vi "dangerEnemy.vi"(8 "error in (no error)":errorcluster, 10 "Game":refnum<class "Game.lvclass">, 11 "Utilities in":refnum<class "Utilities.lvclass">) -> (0 "error out":errorcluster, 2 "Id do Inimigo Mais Próximo":u32, 3 "Utilities out":refnum<class "Utilities.lvclass">, 4 "id do segundo inimigo mais perigoso":i32, 5 "id do inimigo\nmais perigoso":i32, 6 "Pos do segundo inimigo\nperigoso":dbl[](array[numeric]), 7 "Pos do inimigo\nmais perigoso":dbl[](array[numeric]))   [LabVIEW 2018, in "Utilities.lvclass"]
uses:
  Utilities.lvclass
  Game_class/Game.lvclass
  Game_class/Game.lvclass/Game.ctl
  Referee_class/Referee.lvclass/Referee.ctl
  Team_class/Team.lvclass/Team.ctl
  Object_class/Object.lvclass/Object.ctl
  Robot_class/Robot.lvclass/Robot.ctl
  Object_class/Read x.vi
  Object_class/Read y.vi
  Robot_class/Read id.vi
  <vilib>/Analysis/_algsub.llb/Real Vector Norm.vi
  Game_class/Read Referee.vi
  Game_class/Read FieldRef.vi
  Game_class/Read EnemyRef.vi
  Game_class/Read BallRef.vi
  Team_class/Read RobotRef.vi
  Referee_class/Read enemy_goalie_id.vi
  Enemy_class/Enemy.lvclass
  C:/Users/Ronaldo/Desktop/Phoenix/SSL_AI/Team_class/Team.lvclass
  Ball_class/Ball.lvclass
  C:/Users/Ronaldo/Desktop/Phoenix/SSL_AI/Object_class/Object.lvclass
  Robot_class/Robot.lvclass
  Referee_class/Referee.lvclass
  Field_class/Field.lvclass
  <vilib>/Analysis/NI_AALPro.lvlib
panel:
  out "Numero de inimigos\npossiveis para marcar":i32
  in  "D para nao marcar":dbl=200.0
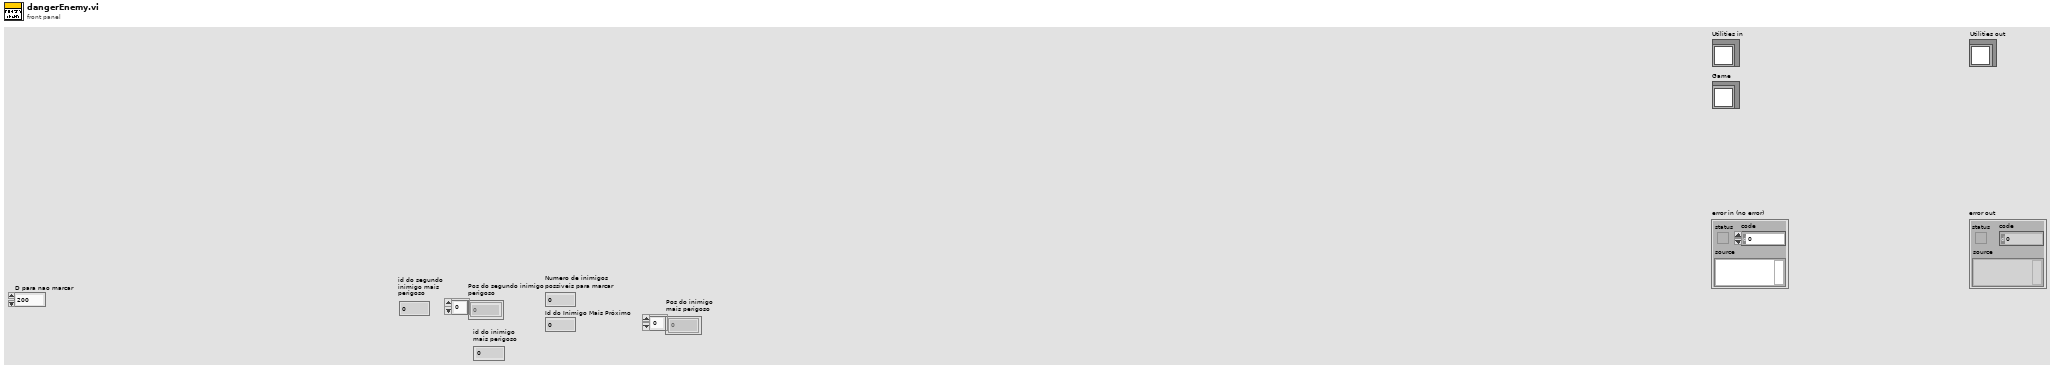
[diagram p1: front panel]
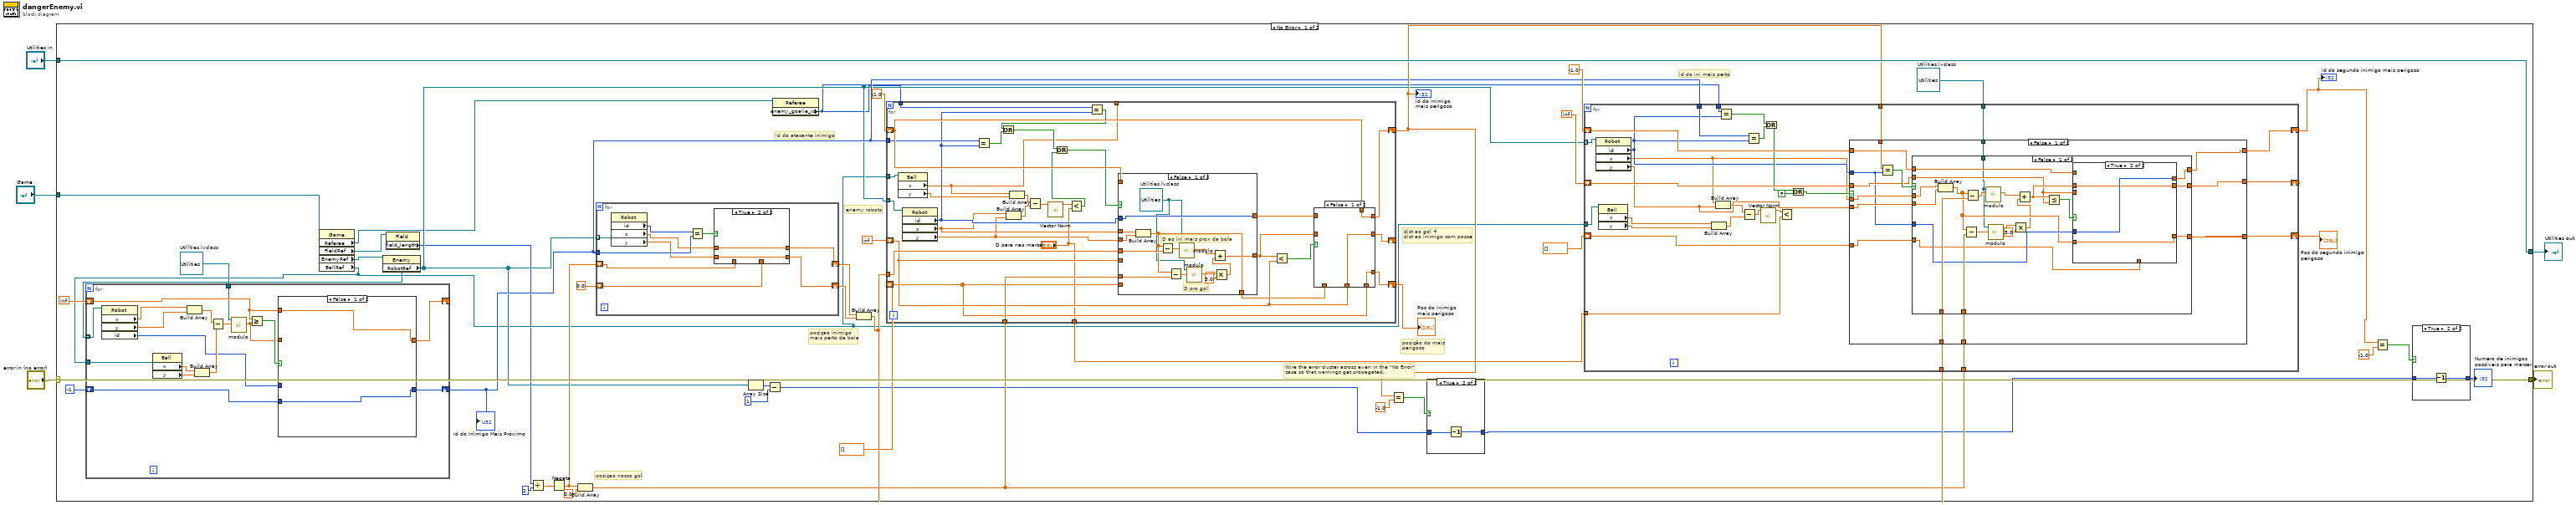
[diagram p0: block diagram]
diagram:
  n1 = case shown="No Error" "error in (no error)" {
    selector: "error in (no error)" -> [w48 w222]
    tunnel: [w48 w222] -> w4
    tunnel: [w49 w221] -> w2
    tunnel: "Utilities in" -> [w49 w221]
    tunnel: "Game" -> [w13 _]
    frame No Error {
      w14 = refnum<class "Utilities.lvclass"> refnum  # Utilities.lvclass
      w15 = refnum<class "Utilities.lvclass"> refnum  # Utilities.lvclass
      # "id do ini mais perto"
      # "id do atacante inimigo"
      # "enemy robots"
      # "dist ao gol +\ndist ao inimigo com posse"
      # "posição do mais\nperigoso"
      # "posiçao nosso gol"
      # "posiçao inimigo\nmais perto da bola"
      # "Wire the error cluster across even in the \"No Error\"\ncase so that warnings get propagated."
      n2 = property class="Game"(reference=w13) -> ("Referee"=w7:refnum<class "Referee.lvclass">, "FieldRef"=w9:refnum<class "Field.lvclass">, "EnemyRef"=w12:refnum<class "Enemy.lvclass">, "BallRef"=w10:refnum<class "Ball.lvclass">)  [unwired: 1 in, 2 out]
      n3 = property class="Enemy"(reference=w12) -> ("RobotRef"=w11:refnum<class "Robot.lvclass">[])  [unwired: 1 in, 2 out]
      n4 = for {
        shift-right: [w67] -> _
        shift-left: inf -> [w65]
        shift-right: [w66] -> w17
        shift-left: -1 -> [w64]
        tunnel: w15 -> [w63]
        tunnel: w10 -> [w62]
        tunnel: w11 -> [w59] mode=indexing
        n5 = property class="Robot"(reference=w59) -> ("x"=w58:dbl, "y"=w57:dbl, "id"=w56:i32)  [unwired: 1 in, 2 out]
        n6 = property class="Ball"(reference=w62) -> ("x"=w61:dbl, "y"=w60:dbl)  [unwired: 1 in, 2 out]
        n7 = Build Array(w58, w57) -> (w72:dbl[])
        n8 = Build Array(w61, w60) -> (w71:dbl[])
        n9 = Subtract(x=w72, y=w71) -> (x-y=w69:dbl[])
        n10 = call "modulo.vi"("2D vector"=w69, "Utilities in"=w63) -> ("Modulo"=w68:dbl)  [unwired: 7 in, 2 out]
        n11 = Greater Or Equal?(x=w65, y=w68) -> (x >= y?=w70:bool)
        n12 = case shown="False" w70 {
          tunnel: [w74 w76] -> w67
          tunnel: w68 -> [_ w76]
          tunnel: w56 -> [_ w75]
          tunnel: [w73 w75] -> w66
          tunnel: w65 -> [w74 _]
          tunnel: w64 -> [w73 _]
          frame False {
          }
          frame True {
          }
        }
      }
      "Id do Inimigo Mais Próximo" <- w17
      n13 = property class="Field"(reference=w9) -> ("field_length"=w8:i32)  [unwired: 1 in, 2 out]
      n14 = Divide(x=w8, y=u32 2) -> (x/y=w45:dbl)
      n15 = Negate(x=w45) -> (-x=w40:dbl)
      n16 = Build Array(w40, 0.0 ("element")) -> (w34:dbl[])
      n17 = for {
        tunnel: w11 -> [w210] mode=indexing
        tunnel: w17 -> [w216]
        shift-right: [w214] -> w19
        shift-left: w40 -> [w212]
        shift-right: [w213] -> w47
        shift-left: 0.0 ("y") -> [w211]
        n18 = property class="Robot"(reference=w210) -> ("id"=w209:i32, "x"=w208:dbl, "y"=w207:dbl)  [unwired: 1 in, 2 out]
        n19 = Equal?(x=w209, y=w216) -> (x = y?=w215:bool)
        n20 = case shown="True" w215 {
          tunnel: w208 -> [_ w220]
          tunnel: w207 -> [_ w219]
          tunnel: [w218 w220] -> w214
          tunnel: [w217 w219] -> w213
          tunnel: w212 -> [w218 _]
          tunnel: w211 -> [w217 _]
          frame False {
          }
          frame True {
          }
        }
      }
      n21 = Array Size(array=w11) -> (size(s)=w31:i32)
      n22 = Subtract(x=w31, y=1) -> (x-y=w26:i32)
      n23 = property class="Referee"(reference=w7) -> ("enemy_goalie_id"=w6:i32)  [unwired: 1 in, 2 out]
      n24 = Build Array(w19, w47) -> (w35:dbl[])
      n25 = for {
        tunnel: w35 -> [w183]
        tunnel: w34 -> [w182]
        shift-right: [w179] -> _
        shift-left: inf -> [w178]
        shift-right: [w176] -> w29
        shift-left: -1.0 ("id") -> [w173]
        shift-right: [w174] -> w43
        shift-left: dbl[] [] -> [w172]
        tunnel: w6 -> [w171]
        tunnel: [w154] -> _
        tunnel: ["D para nao marcar"] -> w20
        tunnel: w17 -> [w161]
        tunnel: w11 -> [w159] mode=indexing
        tunnel: w10 -> [w155]
        n26 = property class="Ball"(reference=w155) -> ("x"=w154:dbl, "y"=w153:dbl)  [unwired: 1 in, 2 out]
        n27 = property class="Robot"(reference=w159) -> ("id"=w158:i32, "x"=w157:dbl, "y"=w156:dbl)  [unwired: 1 in, 2 out]
        n28 = Equal?(x=w161, y=w158) -> (x = y?=w169:bool)
        n29 = Build Array(w157, w156) -> (w167:dbl[])
        n30 = Build Array(w154, w153) -> (w168:dbl[])
        n31 = Subtract(x=w168, y=w167) -> (x-y=w166:dbl[])
        n32 = call-poly <vilib>:"Vector Norm.vi"("Input Vector"=w166) -> ("norm"=w165:dbl)  [unwired: 9 in, 1 out]
        n33 = Less?(x=w165, y="D para nao marcar") -> (x < y?=w160:bool)
        n34 = Equal?(x=w171, y=w158) -> (x = y?=w170:bool)
        n35 = Or(x=w170, y=w169) -> (x .or. y?=w164:bool)
        n36 = Or(x=w164, y=w160) -> (x .or. y?=w163:bool)
        n37 = case shown="False" w163 {
          tunnel: w157 -> [w203 _]
          tunnel: w156 -> [w202 _]
          tunnel: w183 -> [w201 _]
          tunnel: w182 -> [w199 _]
          tunnel: [w196 w206] -> w180
          tunnel: w178 -> [_ w206]
          tunnel: w158 -> [w195 _]
          tunnel: [w195 w205] -> w177
          tunnel: [w194 w204] -> w175
          tunnel: w173 -> [_ w205]
          tunnel: w172 -> [_ w204]
          frame False {
            w190 = refnum<class "Utilities.lvclass"> refnum  # Utilities.lvclass
            # "D ao ini mais prox da bola"
            # "D pro gol"
            n38 = Build Array(w203, w202) -> (w194:dbl[])
            n39 = Subtract(x=w194, y=w201) -> (x-y=w200:dbl[])
            n40 = Subtract(x=w194, y=w199) -> (x-y=w198:dbl[])
            n41 = call "modulo.vi"("2D vector"=w200, "Utilities in"=w190) -> ("Modulo"=w197:dbl)  [unwired: 7 in, 2 out]
            n42 = call "modulo.vi"("2D vector"=w198, "Utilities in"=w190) -> ("Modulo"=w193:dbl)  [unwired: 7 in, 2 out]
            n43 = Multiply(x=w193, y=3.0) -> (x*y=w191:dbl)
            n44 = Add(x=w197, y=w191) -> (x+y=w196:dbl)
          }
          frame True {
          }
        }
        n45 = Less?(x=w180, y=w178) -> (x < y?=w181:bool)
        n46 = case shown="False" w181 {
          tunnel: w180 -> [_ w189]
          tunnel: [w186 w189] -> w179
          tunnel: w178 -> [w186 _]
          tunnel: [w185 w188] -> w176
          tunnel: w177 -> [_ w188]
          tunnel: w173 -> [w185 _]
          tunnel: w175 -> [_ w187]
          tunnel: [w184 w187] -> w174
          tunnel: w172 -> [w184 _]
          frame False {
          }
          frame True {
            # "mais perigoso"
          }
        }
      }
      "id do inimigo\nmais perigoso" <- w29
      "Pos do inimigo\nmais perigoso" <- w43
      n47 = Equal?(x=w29, y=-1.0) -> (x = y?=w27:bool)
      n48 = case shown="True" w27 {
        tunnel: w26 -> [w53 w55]
        tunnel: [w53 w54] -> w22
        frame False {
        }
        frame True {
          n49 = Decrement(x=w55) -> (x-1=w54:i32)
        }
      }
      n50 = for {
        shift-right: [w105] -> w24
        shift-left: -1.0 -> [w104]
        shift-right: [w103] -> _
        shift-left: inf -> [w97]
        shift-right: [w102] -> w36
        shift-left: dbl[] [] -> [w101]
        tunnel: w29 -> [w100]
        tunnel: w35 -> [w99]
        tunnel: w34 -> [w98]
        tunnel: w6 -> [w96]
        tunnel: w20 -> [w89]
        tunnel: w17 -> [w86]
        tunnel: w14 -> [w84]
        tunnel: w11 -> [w83] mode=indexing
        tunnel: w10 -> [w79]
        n51 = property class="Robot"(reference=w83) -> ("id"=w82:i32, "x"=w81:dbl, "y"=w80:dbl)  [unwired: 1 in, 2 out]
        n52 = property class="Ball"(reference=w79) -> ("x"=w78:dbl, "y"=w77:dbl)  [unwired: 1 in, 2 out]
        n53 = Build Array(w78, w77) -> (w92:dbl[])
        n54 = Build Array(w81, w80) -> (w93:dbl[])
        n55 = Equal?(x=w96, y=w82) -> (x = y?=w95:bool)
        n56 = Subtract(x=w93, y=w92) -> (x-y=w91:dbl[])
        n57 = Equal?(x=w86, y=w82) -> (x = y?=w94:bool)
        n58 = call-poly <vilib>:"Vector Norm.vi"("Input Vector"=w91) -> ("norm"=w90:dbl)  [unwired: 9 in, 1 out]
        n59 = Or(x=w95, y=w94) -> (x .or. y?=w88:bool)
        n60 = Less?(x=w90, y=w89) -> ()  [unwired: 1 out]
        n61 = Or(x=w88, y=FALSE) -> (x .or. y?=w87:bool)
        n62 = case shown="False" w87 {
          tunnel: w104 -> [w117 w152]
          tunnel: [w116 w152] -> w105
          tunnel: w97 -> [w115 w151]
          tunnel: [w114 w151] -> w103
          tunnel: w101 -> [w113 w150]
          tunnel: [w112 w150] -> w102
          tunnel: w82 -> [w107 _]
          tunnel: w100 -> [w119 _]
          tunnel: w81 -> [w111 _]
          tunnel: w80 -> [w110 _]
          tunnel: w99 -> [w109 _]
          tunnel: w98 -> [w108 _]
          tunnel: w84 -> [w106 _]
          frame False {
            n63 = Equal?(x=w119, y=w107) -> (x = y?=w118:bool)
            n64 = case shown="False" w118 {
              tunnel: [w132 w149] -> w116
              tunnel: w117 -> [w130 w149]
              tunnel: w115 -> [w124 w148]
              tunnel: [w128 w148] -> w114
              tunnel: w113 -> [w125 w147]
              tunnel: [w126 w147] -> w112
              tunnel: w111 -> [w140 _]
              tunnel: w110 -> [w139 _]
              tunnel: w109 -> [w138 _]
              tunnel: w108 -> [w135 _]
              tunnel: w107 -> [w131 _]
              tunnel: w106 -> [w120 _]
              frame False {
                n65 = Build Array(w140, w139) -> (w127:dbl[])
                n66 = Subtract(x=w127, y=w135) -> (x-y=w134:dbl[])
                n67 = Subtract(x=w127, y=w138) -> (x-y=w137:dbl[])
                n68 = call "modulo.vi"("2D vector"=w137, "Utilities in"=w120) -> ("Modulo"=w136:dbl)  [unwired: 7 in, 2 out]
                n69 = call "modulo.vi"("2D vector"=w134, "Utilities in"=w120) -> ("Modulo"=w123:dbl)  [unwired: 7 in, 2 out]
                n70 = Multiply(x=w123, y=3.0) -> (x*y=w121:dbl)
                n71 = Add(x=w136, y=w121) -> (x+y=w129:dbl)
                n72 = Less Or Equal?(x=w129, y=w124) -> (x <= y?=w133:bool)
                n73 = case shown="True" w133 {
                  tunnel: [w143 w146] -> w132
                  tunnel: w131 -> [_ w146]
                  tunnel: w130 -> [w143 _]
                  tunnel: [w141 w145] -> w128
                  tunnel: w129 -> [_ w145]
                  tunnel: [w142 w144] -> w126
                  tunnel: w127 -> [_ w144]
                  tunnel: w125 -> [w142 _]
                  tunnel: w124 -> [w141 _]
                  frame False {
                  }
                  frame True {
                  }
                }
              }
              frame True {
              }
            }
          }
          frame True {
          }
        }
      }
      "id do segundo inimigo mais perigoso" <- w24
      "Pos do segundo inimigo\nperigoso" <- w36
      n74 = Equal?(x=w24, y=-1.0) -> (x = y?=w23:bool)
      n75 = case shown="True" w23 {
        tunnel: w22 -> [w50 w52]
        tunnel: [w50 w51] -> w21
        frame False {
        }
        frame True {
          n76 = Decrement(x=w52) -> (x-1=w51:i32)
        }
      }
      "Numero de inimigos\npossiveis para marcar" <- w21
    }
    frame Error {
    }
  }
  "error out" <- w4
  "Utilities out" <- w2
